vi "Theoretical BER.vi"(8 "Mapping Parameters":T1={"Modulation Order"=2, "Modulation Type"=0, "Samples per Symbol"=8} {"Modulation Type" items=["PSK", "QAM"]}, 11 "SNRdB":dbl[](array[numeric])) -> (3 "BER":dbl[](array[numeric]))   [LabVIEW 2011]
uses:
  <vilib>/gmath/NI_Gmath.lvlib
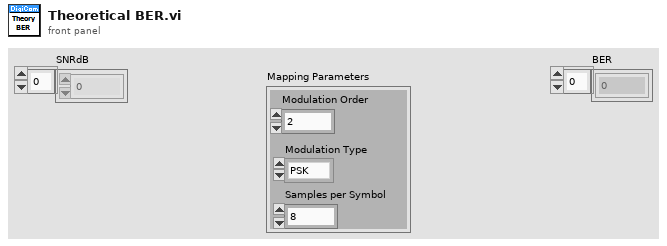
[diagram p1: front panel]
types:
  T1 = cluster{"Modulation Order":i32, "Modulation Type":u16, "Samples per Symbol":i32}
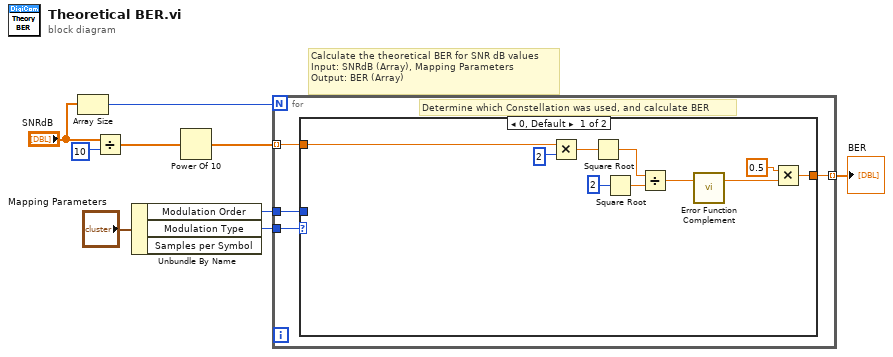
[diagram p0: block diagram]
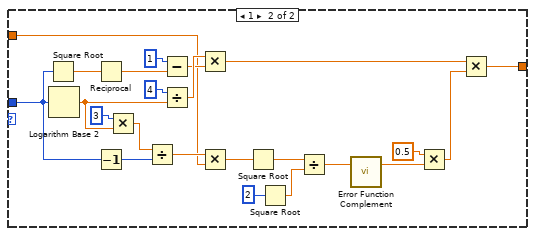
[diagram p2: hidden frame]
diagram:
  # "Calculate the theoretical BER for SNR dB values\nInput: SNRdB (Array), Mapping Parameters\nOutput: BER (Array)"
  n1 = Array Size(array="SNRdB") -> (size(s)=w1:i32)
  n2 = Divide(x="SNRdB", y=10) -> (x/y=w5:dbl[])
  n3 = Unbundle By Name("Mapping Parameters") -> ("Modulation Order"=w7:i32, "Modulation Type"=w8:u16)  [unwired: 1 out]
  n4 = Power Of 10(x=w5) -> (10^x=w4:dbl[])
  n5 = for {
    N: w1 -> [_]
    tunnel: w8 -> [w13]
    tunnel: w7 -> [w12]
    tunnel: w4 -> [w11] mode=indexing
    tunnel: [w10] -> w3 mode=indexing
    # "Determine which Constellation was used, and calculate BER"
    n6 = case shown="0, Default" w13 {
      tunnel: w11 -> [w14 w28]
      tunnel: w12 -> [_ w26]
      tunnel: [w21 w38] -> w10
      frame 0, Default {
        n7 = Multiply(x=w14, y=2) -> (x*y=w16:dbl)
        n8 = Square Root(x=w16) -> (sqrt(x)=w17:dbl)
        n9 = Square Root(x=2) -> (sqrt(x)=w19:dbl)
        n10 = Divide(x=w17, y=w19) -> (x/y=w20:dbl)
        n11 = call <vilib>:"Error Function Complement.vi"("x"=w20) -> ("1 - erf(x)"=w22:dbl)  [unwired: 2 in]
        n12 = Multiply(x=0.5, y=w22) -> (x*y=w21:dbl)
      }
      frame 1 {
        n13 = Square Root(x=w26) -> (sqrt(x)=w34:dbl)
        n14 = Logarithm Base 2(1:w26) -> (0:w27:dbl)
        n15 = Reciprocal(x=w34) -> (1/x=w35:dbl)
        n16 = Decrement(x=w26) -> (x-1=w30:i32)
        n17 = Multiply(x=3, y=w27) -> (x*y=w31:dbl)
        n18 = Divide(x=w31, y=w30) -> (x/y=w29:dbl)
        n19 = Subtract(x=1, y=w35) -> (x-y=w33:dbl)
        n20 = Divide(x=4, y=w27) -> (x/y=w40:dbl)
        n21 = Multiply(x=w40, y=w33) -> (x*y=w39:dbl)
        n22 = Multiply(x=w29, y=w28) -> (x*y=w25:dbl)
        n23 = Square Root(x=w25) -> (sqrt(x)=w24:dbl)
        n24 = Square Root(x=2) -> (sqrt(x)=w43:dbl)
        n25 = Divide(x=w24, y=w43) -> (x/y=w44:dbl)
        n26 = call <vilib>:"Error Function Complement.vi"("x"=w44) -> ("1 - erf(x)"=w45:dbl)  [unwired: 2 in]
        n27 = Multiply(x=0.5, y=w45) -> (x*y=w37:dbl)
        n28 = Multiply(x=w39, y=w37) -> (x*y=w38:dbl)
      }
    }
  }
  "BER" <- w3
